vi "check server.vi"(8 "error in":errorcluster) -> (0 "error out":errorcluster, 2 "timeout?":bool, 4 "Jl Server state out":T3, 5 "return code":u8, 6 "detailed error info":T1)   [LabVIEW 2018, in "LV2Julia_core.lvlib"]
doc: "Pings Julia server, and on success checks the version of the version LabView0mqJl package on the server."
uses:
  LV2Julia_core.lvlib
  Server or client state.ctl
  detailed error info.ctl
  StackFrame.ctl
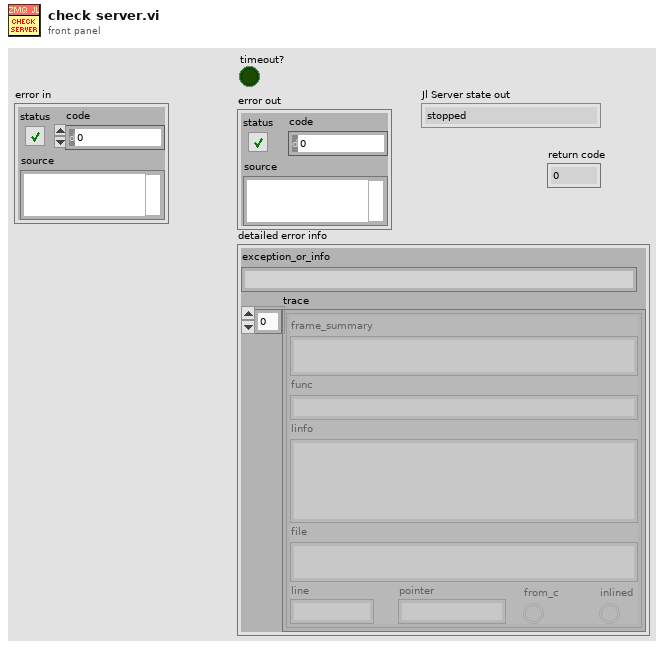
[diagram p1: front panel]
types:
  T1 = typedef "LV2Julia_core.lvlib/detailed error info.ctl" = cluster{"exception_or_info":string, "trace":T2[]}
  T2 = typedef "LV2Julia_core.lvlib/StackFrame.ctl" = cluster{"frame_summary":string, "func":string, "linfo":string, "file":string, "line":i32, "pointer":u64, "from_c":bool, "inlined":bool}
  T3 = typedef "LV2Julia_core.lvlib/Server or client state.ctl" = enum16{"stopped", "running", "unknown"}
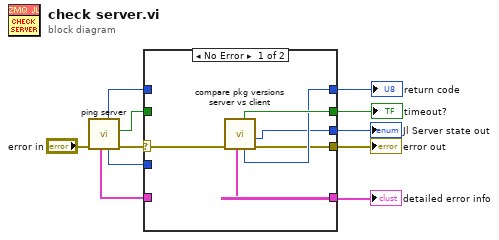
[diagram p0: block diagram]
diagram:
  n1 = call "ping server.vi"("error in"="error in") -> ("error out"=w10:errorcluster, "timeout?"=w1:bool, "Jl Server state out"=w6:T3, "return code"=w3:u8, "detailed error info"=w8:T1)  [unwired: 6 in]
  n2 = case shown="No Error" w10 {
    selector: w10 -> [w17 w22]
    tunnel: [w14 w22] -> w9
    tunnel: [w12 w21] -> w7
    tunnel: w8 -> [_ w21]
    tunnel: [w13 w20] -> w5
    tunnel: w6 -> [_ w20]
    tunnel: [w15 w19] -> w4
    tunnel: w3 -> [_ w19]
    tunnel: [w16 w18] -> w2
    tunnel: w1 -> [_ w18]
    frame No Error {
      n3 = call "compare pkg versions server vs client.vi"("error in (no error)"=w17) -> ("error out"=w14:errorcluster, "Jl Server state out"=w13:T3, "return code"=w15:u8, "timeout?"=w16:bool, "detailed error info"=w12:T1)  [unwired: 4 in, 2 out]
    }
    frame Error {
    }
  }
  "error out" <- w9
  "timeout?" <- w2
  "Jl Server state out" <- w5
  "detailed error info" <- w7
  "return code" <- w4
